vi "CLEventPlayback.vi"() -> ()   [LabVIEW 2017]
uses:
  <vilib>/DAQmx/read.llb/DAQmx Read (Counter U32 1Chan 1Samp).vi
  <vilib>/DAQmx/miscellaneous.llb/DAQmx Fill In Error Info.vi
panel:
  in  "Events file":path
  in  "OEP sample clock in":tag="/pciDAQ/PFI0"
  in  "Onboard counter":tag="pciDAQ/ctr0"
  in  "Digital real/sham stim channels":tag="pciDAQ/port0/line1:2"
  in  "Analog pulse channel":tag="pciDAQ/ao0"
  in  "OEP stim/sham TTL chans":u16[](array[numeric])=[2, 3] caption="probe channel" min=1 max=8
  in  "event port":u16=5557
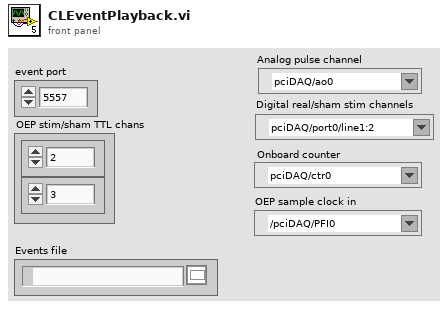
[diagram p1: front panel]
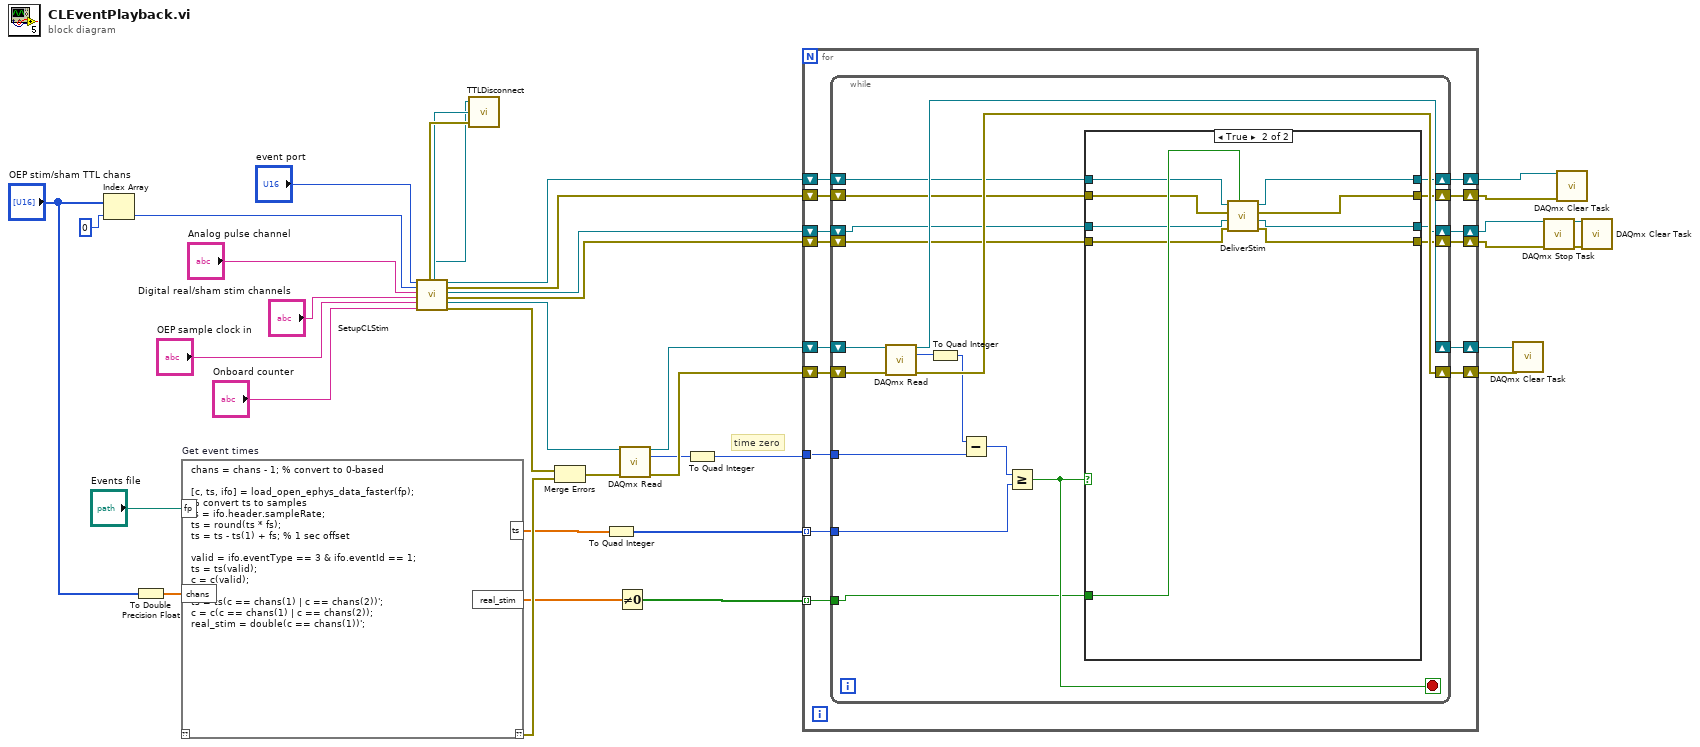
[diagram p0: block diagram]
diagram:
  # "time zero"
  n1 = Index Array(array="OEP stim/sham TTL chans", index=0) -> (element=w35:u16)
  n2 = To Double Precision Float(number="OEP stim/sham TTL chans") -> (double precision float=w33:dbl[])
  n3 = script code="chans = chans - 1; % convert to 0-based\n\n[c, ts, ifo] = load_open_ephys_data_faster(fp);\n% convert ts to samples\nfs = ifo.header.sampleRate;\nts = round(ts * fs);\nts = ts - ts(1) + fs; % 1 sec offset\n\nvalid = ifo.eventType == 3 & ifo.eventId == 1;\nts = ts(valid);\nc = c(valid);\n\nts = ts(c == chans(1) | c == chans(2))';\nc = c(c == chans(1) | c == chans(2));\nreal_stim = double(c == chans(1))';" "Get event times"("fp"="Events file", "chans"=w33) -> ("??"=w3:errorcluster, "ts"=w1:dbl[], "real_stim"=w2:dbl[])  [unwired: 1 in]
  n4 = call "SetupCLStim.vi"("event port"="event port", "OEP pulse channel"=w35, "Analog pulse channel"="Analog pulse channel", "Digital real/sham stim channels"="Digital real/sham stim channels", "OEP sample clock in"="OEP sample clock in", "Onboard counter"="Onboard counter") -> ("zmq error out"=w22:errorcluster, "context out"=w20:refnum<class "zmq_context.lvclass">, "socket out"=w21:refnum<class "zmq_socket.lvclass">, "AO task out"=w17:refnum<k21>, "AO error out"=w16:errorcluster, "DO task out"=w15:refnum<k21>, "DO error out"=w14:errorcluster, "ctr task out"=w26:refnum<k21>, "ctr error out"=w4:errorcluster)  [unwired: 4 in, 1 out]
  n5 = call "TTLDisconnect.vi"("error in"=w22, "socket in"=w21, "context in"=w20) -> ()  [unwired: 1 in, 1 out]
  n6 = Merge Errors(w4, w3) -> (w5:errorcluster)
  n7 = To Quad Integer(1:w1) -> (0:w23:i64[])
  n8 = Not Equal To 0?(x=w2) -> (x != 0?=w27:bool[])
  n9 = call-poly <vilib>:"DAQmx Read.vi"("task/channels in"=w26, "error in"=w5) -> ("task out"=w25:refnum<k21>, "data"=w19:u32, "error out"=w24:errorcluster)  [unwired: 11 in]
  n10 = To Quad Integer(1:w19) -> (0:w18:i64)
  n11 = for {
    tunnel: w27 -> [w47] mode=indexing
    tunnel: w18 -> [w48]
    shift-right: [w50] -> w7
    shift-left: w25 -> [w52]
    shift-right: [w49] -> w6
    shift-left: w24 -> [w51]
    tunnel: w23 -> [w46] mode=indexing
    shift-right: [w41] -> w11
    shift-left: w17 -> [w45]
    shift-right: [w40] -> w10
    shift-left: w16 -> [w44]
    shift-right: [w38] -> w8
    shift-left: w14 -> [w42]
    shift-right: [w39] -> w9
    shift-left: w15 -> [w43]
    n12 = while {
      shift-right: [w69] -> w50
      shift-left: w52 -> [w71]
      shift-right: [w68] -> w49
      shift-left: w51 -> [w70]
      tunnel: w48 -> [w67]
      tunnel: w47 -> [w61]
      tunnel: w46 -> [w63]
      shift-right: [w56] -> w41
      shift-left: w45 -> [w60]
      shift-right: [w55] -> w40
      shift-left: w44 -> [w59]
      shift-right: [w54] -> w39
      shift-left: w43 -> [w58]
      shift-right: [w53] -> w38
      shift-left: w42 -> [w57]
      stop <- w62 stop-if-true
      n13 = call-poly <vilib>:"DAQmx Read.vi"("task/channels in"=w71, "error in"=w70) -> ("task out"=w69:refnum<k21>, "data"=w66:u32, "error out"=w68:errorcluster)  [unwired: 11 in]
      n14 = To Quad Integer(1:w66) -> (0:w65:i64)
      n15 = Subtract(x=w65, y=w67) -> (x-y=w64:i64)
      n16 = Greater Or Equal?(x=w64, y=w63) -> (x >= y?=w62:bool)
      n17 = case shown="True" w62 {
        tunnel: w61 -> [_ w84]
        tunnel: w60 -> [w75 w83]
        tunnel: w59 -> [w74 w82]
        tunnel: w58 -> [w73 w81]
        tunnel: w57 -> [w72 w80]
        tunnel: [w75 w79] -> w56
        tunnel: [w74 w78] -> w55
        tunnel: [w73 w77] -> w54
        tunnel: [w72 w76] -> w53
        frame False {
        }
        frame True {
          n18 = call "DeliverStim.vi"("Real stim on"=w84, "DO error in"=w80, "DO task in"=w81, "AO error in"=w82, "AO task in"=w83) -> ("DO error out"=w76:errorcluster, "DO task out"=w77:refnum<k21>, "AO error out"=w78:errorcluster, "AO task out"=w79:refnum<k21>)
        }
      }
    }
  }
  n19 = call <vilib>:"DAQmx Clear Task.vi"("task in"=w7, "error in"=w6) -> ()  [unwired: 13 in, 1 out]
  n20 = call <vilib>:"DAQmx Stop Task.vi"("task/channels in"=w9, "error in"=w8) -> ("task out"=w12:refnum<k21>, "error out"=w13:errorcluster)  [unwired: 12 in]
  n21 = call <vilib>:"DAQmx Clear Task.vi"("task in"=w11, "error in"=w10) -> ()  [unwired: 13 in, 1 out]
  n22 = call <vilib>:"DAQmx Clear Task.vi"("task in"=w12, "error in"=w13) -> ()  [unwired: 13 in, 1 out]
